vi "GEA3 COM Port Check.vi"() -> ()   [LabVIEW 2023]
uses:
  library/GEA2_Toolkit.lvlib
panel:
  out "Message":string
  out "Board ID":string
  out "COM Port":string
  # "COM Port Check"
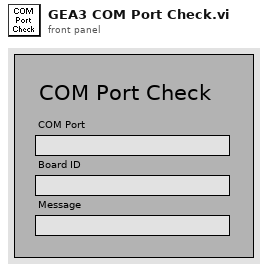
[diagram p1: front panel]
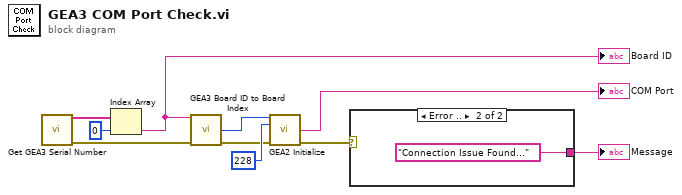
[diagram p0: block diagram]
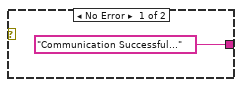
[diagram p2: hidden frame]
diagram:
  n1 = call "Get GEA3 Serial Number.vi"() -> ("GEA3 Serial Numbers"=w9:string[], "Error Out"=w8:errorcluster)  [unwired: 14 in]
  n2 = Index Array(array=w9, index=0) -> (element=w3:string)
  "Board ID" <- w3
  n3 = call "GEA3 Board ID to Board Index.vi"("GEA3 Serial Number"=w3, "Error In"=w8) -> ("Board Index"=w7:i32, "Error Out"=w6:errorcluster)  [unwired: 9 in, 3 out]
  n4 = call "GEA2 Initialize.vi"("Board Index"=w7, "Source Address"=u8 228, "error in"=w6) -> ("Board ID"=→"COM Port":string, "error out"=w2:errorcluster)  [unwired: 10 in, 1 out]
  n5 = case shown="Error .." w2 {
    tunnel: ["Communication Successful..." "Connection Issue Found..."] -> w1
    frame No Error {
    }
    frame Error {
    }
  }
  "Message" <- w1
